vi "PCANTerminal.vi"() -> ()   [LabVIEW 2020]
panel:
  out "Time()":u32
  out "Message":string[](array[string])
  out "次数":i32[](array[numeric])
  in  "Transmit":T1(array[cluster])=[{"ID"=828, "MSGTYPE"=0, "LEN"=8, "Data"=[2, 0, 0, 0, 0, 0, 0, 0], "Time"=100}, {"ID"=860, "MSGTYPE"=0, "LEN"=8, "Data"=[20, 0, 169, 128, 74, 148, 160, 9], "Time"=100}, {"ID"=917, "MSGTYPE"=0, "LEN"=8, "Data"=[0, 0, 0, 0, 0, 0, 0, 0], "Time"=100}, {"ID"=1409, "MSGTYPE"=0, "LEN"=8, "Data"=[129, 0, 0, 0, 0, 0, 0, 0], "Time"=500}, {"ID"=911, "MSGTYPE"=0, "LEN"=8, "Data"=[0, 0, 8, 0, 0, 0, 0, 0], "Time"=100}] {"ID" format="%.0x"; "MSGTYPE" items=["STATUS"=128, "EXTENDED"=2, "RTR"=1, "DATA MSG"=0]; "Data" format="%.2x"}
  out "TPCANMsg 2":T2(array[cluster]) {"ID" format="%.0x"; "aDATA" format="%.0x"}
  in  "停止":bool
  out "LastError":string
  out "TPCANMsg":T3 {"ID" format="%.0x"; "aDATA" format="%.0x"}
  out "Version":string
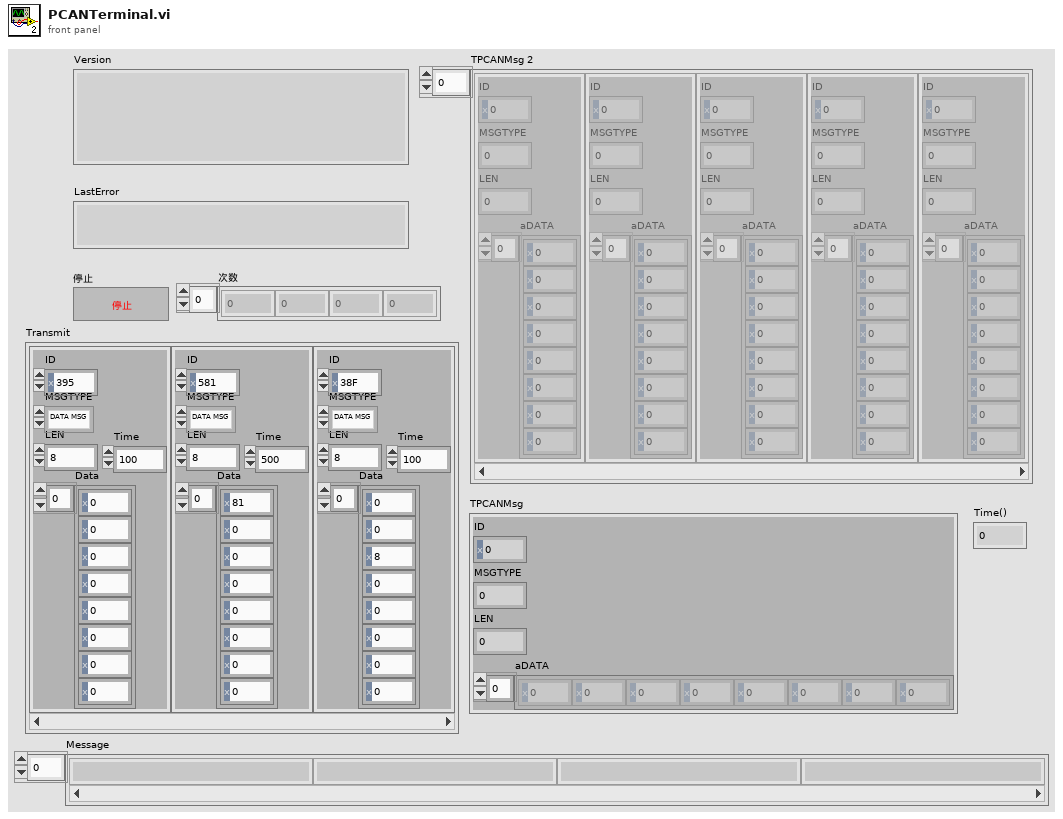
[diagram p1: front panel]
types:
  T1 = cluster{"ID":u32, "MSGTYPE":u8, "LEN":u8, "Data":u8[], "Time":u16}[]
  T2 = cluster{"ID":u32, "MSGTYPE":u8, "LEN":u8, "aDATA":u8[]}[]
  T3 = cluster{"ID":u32, "MSGTYPE":u8, "LEN":u8, "aDATA":u8[]}
  T4 = cluster{"Is Warning":bool, "Is Error":bool, "Message":string}
  T5 = cluster{"ID":u32, "MSGTYPE":u8, "LEN":u8, "Data":u8[]}[]
  T6 = cluster{"ID":u32, "MSGTYPE":u8, "LEN":u8, "Data":u8[]}
  T7 = cluster{"Time":u16, "MessageBuffer":cluster{"ID":u32, "MSGTYPE":u8, "LEN":u8, "DATA[0]":u8, "DATA[1]":u8, "DATA[2]":u8, "DATA[3]":u8, "DATA[4]":u8, "DATA[5]":u8, "DATA[6]":u8, "DATA[7]":u8}[]}[]
  T8 = typedef "PCAN_ERROR.ctl" = i32
  T9 = cluster{"ID":u32, "MSGTYPE":u8, "LEN":u8, "DATA[0]":u8, "DATA[1]":u8, "DATA[2]":u8, "DATA[3]":u8, "DATA[4]":u8, "DATA[5]":u8, "DATA[6]":u8, "DATA[7]":u8}[]
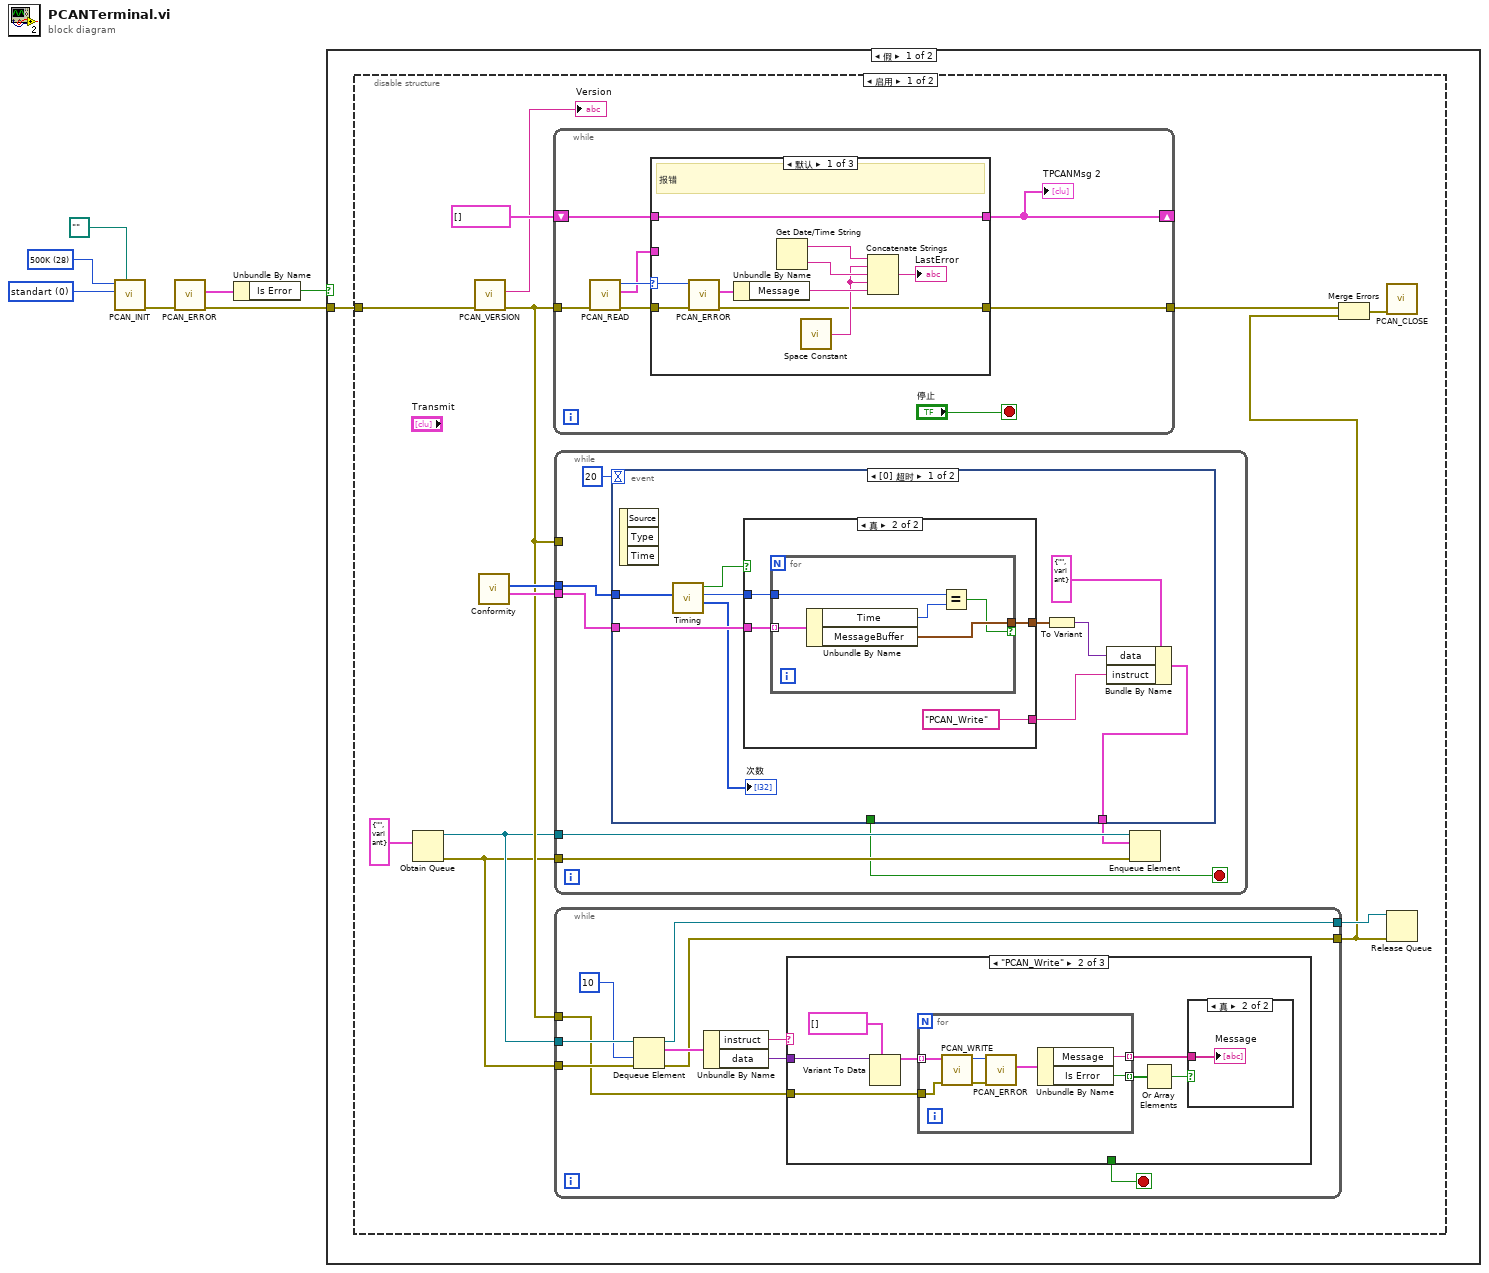
[diagram p0: block diagram]
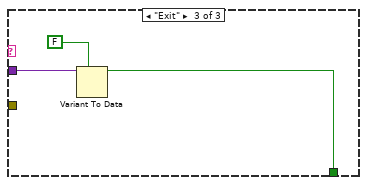
[diagram p4: hidden frame]
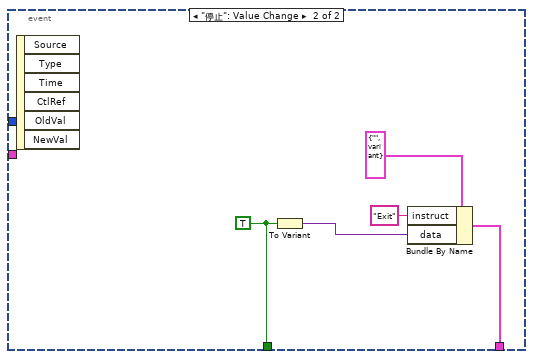
[diagram p6: hidden frame]
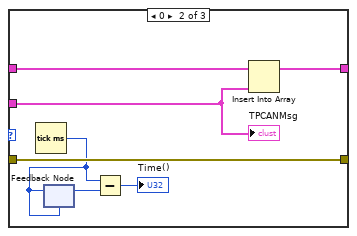
[diagram p7: hidden frame]
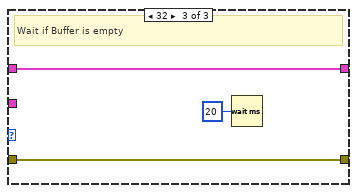
[diagram p8: hidden frame]
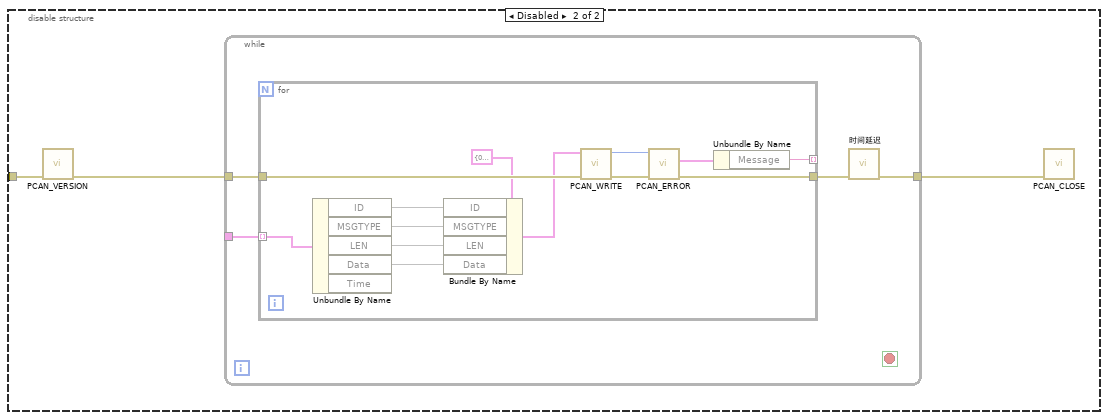
[diagram p9: hidden frame]
diagram:
  w6 = 0 items=["standart", "extended"] ("Msg Type")
  w7 = u16 28 items=["1M"=20, "500K"=28, "250K"=284, "125K"=796, "100K"=17199, "50K"=18223, "20K"=21295, "10K"=26415, "5K"=32639] ("BTR0BTR1")
  n1 = call <userlib>:"PCAN_INIT.vi"("path in"=path "", "Msg Type"=w6, "BTR0BTR1"=w7) -> ("error out"=w5:errorcluster)  [unwired: 6 in, 2 out]
  n2 = call <userlib>:"PCAN_ERROR.vi"("error in (no error)"=w5) -> ("error out"=w2:errorcluster, "PCAN error"=w4:T4)  [unwired: 8 in, 1 out]
  n3 = Unbundle By Name(w4) -> ("Is Error"=w3:bool)
  n4 = case shown="假" w3 {
    tunnel: w2 -> [w8 _]
    frame False {
      n5 = disable-structure shown="启用" {
        disable-tunnel: w8 -> [w21 w111]
        frame Enabled {
          n6 = Obtain Queue(element data type=cluster{"instruct":string, "data":variant} {"instruct"="", "data"=variant}) -> (queue out=w15:refnum<queue>, error out=w14:errorcluster)  [unwired: 4 in, 1 out]
          n7 = call <userlib>:"PCAN_VERSION.vi"("error in (no error)"=w21) -> ("error out"=w17:errorcluster, "lpszTextBuff"=→"Version":string)  [unwired: 7 in, 2 out]
          n8 = call "Conformity.vi"() -> ("整合后"=w18:T7, "时间段"=w19:u16[])  [unwired: 10 in]
          n9 = while {
            tunnel: w17 -> [w88]
            tunnel: [w84] -> w11
            shift-right: [w82] -> _
            shift-left: T2 [] -> [w83]
            stop <- "停止" stop-if-true
            n10 = call <userlib>:"PCAN_READ.vi"("error in (no error)"=w88) -> ("error out"=w87:errorcluster, "TPCANMsg"=w85:T3, "error"=w86:T8)  [unwired: 7 in, 1 out]
            n11 = case shown="默认" w86 {
              selector: w86 -> [w97 _ _]
              tunnel: w87 -> [w98 w105 w108]
              tunnel: w85 -> [_ w104 _]
              tunnel: [w90 w105 w108] -> w84
              tunnel: [w89 w103 w106] -> w82
              tunnel: w83 -> [w89 w102 w106]
              frame Default {
                # "报错"
                n12 = call <userlib>:"PCAN_ERROR.vi"("error in (no error)"=w98, "Error Code"=w97) -> ("error out"=w90:errorcluster, "PCAN error"=w96:T4)  [unwired: 7 in, 1 out]
                n13 = Unbundle By Name(w96) -> ("Message"=w93:string)
                n14 = Get Date/Time String() -> (date string=w95:string, time string=w94:string)  [unwired: 3 in]
                n15 = call <vilib>:"Space Constant.vi"() -> ("String"=w92:string)
                n16 = Concatenate Strings(w95, w92, w94, w92, w93) -> (→"LastError":string)
              }
              frame 0 {
                n17 = Tick Count (ms)() -> (millisecond timer value=w100:u32)
                n18 = feedback-in #1(w100) -> ()
                n19 = feedback #1(w100) -> (w101:u32)
                n20 = Subtract(x=w100, y=w101) -> (x-y=→"Time()":u32)
                n21 = Insert Into Array(array=w102, new element=w104) -> (w103:T2)  [unwired: 1 in]
                "TPCANMsg" <- w104
              }
              frame 32 {
                # "Wait if Buffer is empty"
                n22 = Wait (ms)(milliseconds to wait=u32 20 ("等待时间（毫秒）")) -> ()  [unwired: 1 out]
              }
            }
            "TPCANMsg 2" <- w82
          }
          n23 = while {
            tunnel: w17 -> [_]
            tunnel: w19 -> [w56]
            tunnel: w18 -> [w55]
            tunnel: w15 -> [w54]
            tunnel: w14 -> [w53]
            stop <- w50 stop-if-true
            n24 = event shown="[0] 超时" {
              selector: _ -> [_ _]
              dyn-events: _ -> [_ _]
              timeout: 20 -> [_ _]
              tunnel: w56 -> [w66 _]
              tunnel: w55 -> [w63 _]
              tunnel: [w58 w77] -> w52
              tunnel: [_ w76] -> w50
              event Timeout {
                n25 = event-data() -> ()  [unwired: 1 in, 3 out]
                n26 = call "Timing.vi"("数组"=w66) -> ("次数"=→"次数":i32[], "当前"=w64:u16, "到"=w65:bool)  [unwired: 8 in]
                n27 = case shown="真" w65 {
                  tunnel: w64 -> [_ w69]
                  tunnel: w63 -> [_ w70]
                  tunnel: [_ w68] -> w61
                  tunnel: [_ "PCAN_Write"] -> w57
                  frame False {
                  }
                  frame True {
                    n28 = for {
                      tunnel: w70 -> [w75] mode=indexing
                      tunnel: w69 -> [w73]
                      tunnel: [w72] -> w68 if=w71
                      n29 = Unbundle By Name(w75) -> ("Time"=w74:u16, "MessageBuffer"=w72:T9)
                      n30 = Equal?(x=w73, y=w74) -> (x = y?=w71:bool)
                    }
                  }
                }
                n31 = To Variant(anything=w61) -> (Variant=w59:variant)
                n32 = Bundle By Name(cluster=cluster{"instruct":string, "data":variant} {"instruct"="", "data"=variant}, "data"=w59, "instruct"=w57) -> (w58:cluster{"instruct":string, "data":variant})
              }
              event "停止": Value Change {
                w76 = TRUE
                n33 = event-data() -> ()  [unwired: 1 in, 6 out]
                n34 = To Variant(anything=w76) -> (Variant=w78:variant)
                n35 = Bundle By Name(cluster=cluster{"instruct":string, "data":variant} {"instruct"="", "data"=variant}, "instruct"="Exit", "data"=w78) -> (w77:cluster{"instruct":string, "data":variant})
              }
            }
            n36 = Enqueue Element(queue=w54, element=w52, error in (no error)=w53) -> ()  [unwired: 1 in, 3 out]
          }
          n37 = while {
            tunnel: w17 -> [w25]
            tunnel: w15 -> [w31]
            tunnel: w14 -> [w30]
            tunnel: [w23] -> w13
            tunnel: [w22] -> w10
            stop <- w24 stop-if-true
            n38 = Dequeue Element(queue=w31, timeout in ms (-1)=10 ("超时毫秒(-1)"), error in (no error)=w30) -> (queue out=w23:refnum<queue>, element=w28:cluster{"instruct":string, "data":variant}, error out=w22:errorcluster)  [unwired: 1 out]
            n39 = Unbundle By Name(w28) -> ("instruct"=w27:string, "data"=w26:variant)
            n40 = case shown="\"PCAN_Write\"" w27 {
              tunnel: w26 -> [_ w38 w49]
              tunnel: w25 -> [_ w35 _]
              tunnel: [_ _ w47] -> w24
              frame "", Default {
              }
              frame "PCAN_Write" {
                n41 = Variant To Data(type=T5 [] ("TPCANMsg"), Variant=w38) -> (data=w36:T5)  [unwired: 1 in, 1 out]
                n42 = for {
                  tunnel: w36 -> [w46] mode=indexing
                  tunnel: w35 -> [w45]
                  tunnel: [w41] -> w32 mode=indexing
                  tunnel: [w40] -> w34 mode=indexing
                  n43 = call <userlib>:"PCAN_WRITE.vi"("error in (no error)"=w45, "TPCANMsg"=w46) -> ("error out"=w43:errorcluster, "error"=w44:T8)  [unwired: 7 in, 1 out]
                  n44 = call <userlib>:"PCAN_ERROR.vi"("error in (no error)"=w43, "Error Code"=w44) -> ("PCAN error"=w42:T4)  [unwired: 7 in, 2 out]
                  n45 = Unbundle By Name(w42) -> ("Message"=w41:string, "Is Error"=w40:bool)
                }
                n46 = Or Array Elements(Boolean array=w34) -> (logical OR=w33:bool)
                n47 = case shown="真" w33 {
                  tunnel: w32 -> [_ w39]
                  frame False {
                  }
                  frame True {
                    "Message" <- w39
                  }
                }
              }
              frame "Exit" {
                n48 = Variant To Data(type=FALSE, Variant=w49) -> (data=w47:bool)  [unwired: 1 in, 1 out]
              }
            }
          }
          n49 = Merge Errors(w11, w10) -> (w9:errorcluster)
          n50 = call <userlib>:"PCAN_CLOSE.vi"("error in (no error)"=w9) -> ()  [unwired: 9 in, 2 out]
          n51 = Release Queue(queue=w13, error in (no error)=w10) -> ()  [unwired: 1 in, 3 out]
        }
        frame Disabled {
          n52 = call <userlib>:"PCAN_VERSION.vi"("error in (no error)"=w111) -> ("error out"=w110:errorcluster)  [unwired: 7 in, 3 out]
          n53 = while {
            tunnel: w110 -> [w115]
            tunnel: _ -> [w114]
            tunnel: [w112] -> w109
            stop <- _ stop-if-true
            n54 = for {
              tunnel: w115 -> [w128]
              tunnel: w114 -> [w127] mode=indexing
              tunnel: [w117] -> _ mode=indexing
              tunnel: [w116] -> w113
              n55 = Unbundle By Name(w127) -> ("ID"=w125, "MSGTYPE"=w124, "LEN"=w123, "Data"=w122)  [unwired: 1 out]
              n56 = Bundle By Name(cluster=T6 {"ID"=0, "MSGTYPE"=128, "LEN"=0, "Data"=[]} ("TPCANMsg"), "ID"=w125, "MSGTYPE"=w124, "LEN"=w123, "Data"=w122) -> (w121:T6)
              n57 = call <userlib>:"PCAN_WRITE.vi"("error in (no error)"=w128, "TPCANMsg"=w121) -> ("error out"=w120:errorcluster, "error"=w119:T8)  [unwired: 7 in, 1 out]
              n58 = call <userlib>:"PCAN_ERROR.vi"("error in (no error)"=w120, "Error Code"=w119) -> ("error out"=w116:errorcluster, "PCAN error"=w118:T4)  [unwired: 7 in, 1 out]
              n59 = Unbundle By Name(w118) -> ("Message"=w117:string)
            }
            n60 = call "时间延迟"("error in (no error)"=w113) -> ("error out"=w112:errorcluster)  [unwired: 10 in]
          }
          n61 = call <userlib>:"PCAN_CLOSE.vi"("error in (no error)"=w109) -> ()  [unwired: 9 in, 2 out]
        }
      }
    }
    frame True {
    }
  }
